vi "Temp_sub_VI_Peltier control exzample PID.vi"(11 "mean":dbl) -> (3 "T":dbl)   [LabVIEW 2013]
uses:
  <vilib>/express/express arith-compare/Formula/XNode/ExpressFormulaBlockNode.xnode
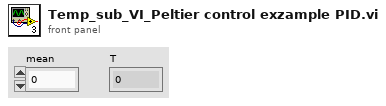
[diagram p1: front panel]
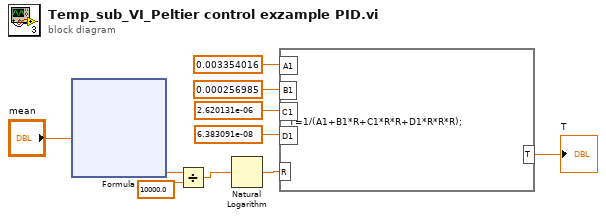
[diagram p0: block diagram]
diagram:
  n1 = xnode "Formula"("V"="mean") -> ("Result"=w1:dbl)  [unwired: 1 in, 1 out]
  n2 = Divide(x=w1, y=10000.0) -> (x/y=w4:dbl)
  n3 = Natural Logarithm(1:w4) -> (0:w2:dbl)
  n4 = formula code="T=1/(A1+B1*R+C1*R*R+D1*R*R*R);"("R"=w2, "A1"=0.003354016 ("input variable"), "B1"=0.000256985 ("input variable"), "C1"=2.620131e-06 ("input variable"), "D1"=6.383091e-08 ("input variable")) -> ("T"=→"T":dbl)
